vi "Voltage and Current Ring Chooser.vi"(8 "error in (no error)":errorcluster, 11 "Yokogawa WT1600 in":refnum<class "Yokogawa WT1600.lvclass">) -> (0 "error out":errorcluster, 3 "Yokogawa WT1600 out":refnum<class "Yokogawa WT1600.lvclass">)   [LabVIEW 2016, in "Generic Power Analyzer.lvlib" / "Yokogawa WT1600.lvlib" / "Yokogawa WT1600.lvclass"]
uses:
  Yokogawa WT1600.lvclass
panel:
  in  "A Range (9: 5A)":u16(ring)=9 items=["AUTO", "10 mA", "20 mA", "50 mA", "100 mA", "200 mA", "500 mA", "1 A", "2 A", "5 A", "10 A", "20 A", "50 A", "S-AUTO", "50 mV", "100 mV", "250 mV", "500 mV", "1 V", "2.5 V", "5 V", "10 V"]
  in  "V Range (12: 1000)":u16(ring)=12 items=["AUTO", "1.5", "3", "6", "10", "15", "30", "60", "100", "150", "300", "600", "1000"]
  in  "Wiring A (0: 1P2W)":u16(ring) items=["1P2W", "1P3W", "3P3W", "3P4W", "3V3A"]
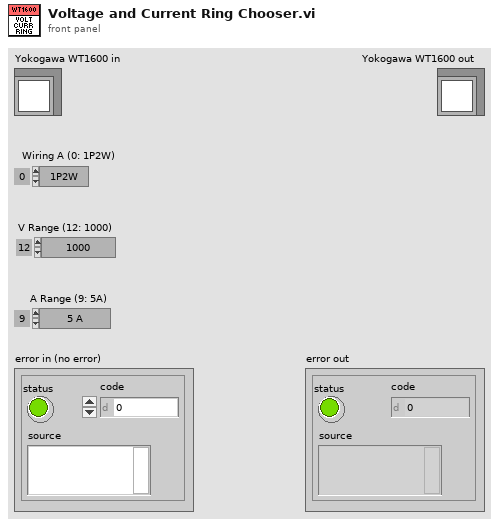
[diagram p1: front panel]
types:
  T1 = typedef "LVStringsAndValuesArrayTypeDef_U16.ctl" = cluster{"String":string, "Value":u16}[]
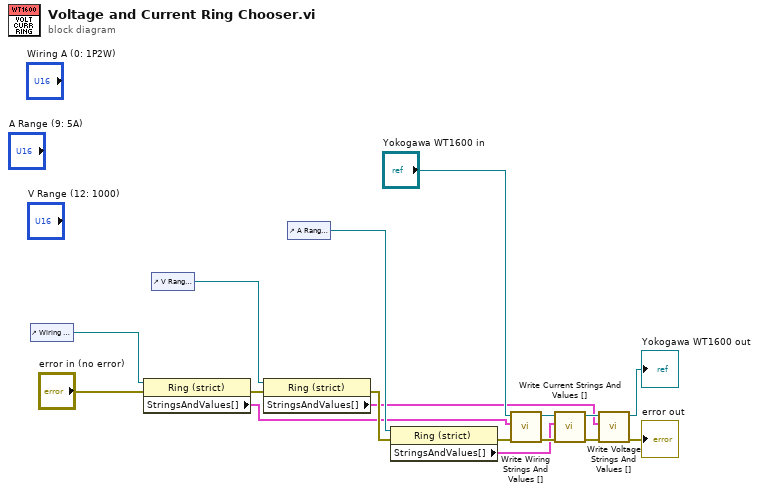
[diagram p0: block diagram]
diagram:
  n1 = control-ref of="Wiring A (0: 1P2W)"() -> (w17:refnum<vi>)
  n2 = property class="Ring (strict)"(reference=w17, error in="error in (no error)") -> (error out=w7:errorcluster, "StringsAndValues[]"=w3:T1)  [unwired: 1 out]
  n3 = control-ref of="V Range (12: 1000)"() -> (w8:refnum<vi>)
  n4 = property class="Ring (strict)"(reference=w8, error in=w7) -> (error out=w6:errorcluster, "StringsAndValues[]"=w2:T1)  [unwired: 1 out]
  n5 = control-ref of="A Range (9: 5A)"() -> (w9:refnum<vi>)
  n6 = property class="Ring (strict)"(reference=w9, error in=w6) -> (error out=w4:errorcluster, "StringsAndValues[]"=w1:T1)  [unwired: 1 out]
  n7 = call-dynamic "Write Wiring Strings And Values [].vi"("error in (no error)"=w4, "Strings And Values []"=w3, "Generic Power Analyzer in"="Yokogawa WT1600 in") -> ("error out"=w12:errorcluster, "Generic Power Analyzer out"=w15:refnum<class "Yokogawa WT1600.lvclass">)  [unwired: 7 in]
  n8 = call-dynamic "Write Current Strings And Values [].vi"("error in (no error)"=w12, "Strings And Values []"=w1, "Generic Power Analyzer in"=w15) -> ("error out"=w11:errorcluster, "Generic Power Analyzer out"=w14:refnum<class "Yokogawa WT1600.lvclass">)  [unwired: 7 in]
  n9 = call-dynamic "Write Voltage Strings And Values [].vi"("error in (no error)"=w11, "Strings And Values []"=w2, "Generic Power Analyzer in"=w14) -> ("error out"=→"error out":errorcluster, "Generic Power Analyzer out"=→"Yokogawa WT1600 out":refnum<class "Yokogawa WT1600.lvclass">)  [unwired: 7 in]
